vi "young.vi"() -> ()   [LabVIEW 2018]
doc: "Logs and displays weather data in real-time from the Vaisala WXT520 Weather Station and the Optical Scientific ORG-815 Optical Rain Gauge."
uses:
  <vilib>/Analysis/baseanly.llb/Mean (DBL).vi
  <vilib>/Platform/browser.llb/Open URL in Default Browser (path).vi
  <vilib>/Analysis/NI_AALBase.lvlib
panel:
  out "Wind Gusts":dbl format="%.3g"
  out "RF Propagation Logo":picture
  in  "Show Legend":bool
  out "Young Logo":picture
  in  "Young Prefix":string="Young"
  in  "Young":refnum<visa-resource-name>="Port3"
  out "Date":string="2012/06/22\n12:33:20 PM"
  out "Wind Direction":dbl format="%.3g"
  out "Wind Speed":dbl format="%.3g"
  out "Pressure":dbl format="%.3g"
  out "Humidity":dbl format="%.3g"
  out "Temperature":dbl format="%.3g"
  in  "Open Output":bool
  out "Running LED":bool
  out "Uptime":string="00:00:00"
  out "Progress Bar":u32(slide) scale=0.0..60.0
  in  "stop":bool
  out "Timestamp":dbl
  in  "Output Path":path=path "C:/Users/Bruce Wayne/Desktop/DELETE_WeatherTest"
  out "Rain Fall":dbl format="%.3g"
  out "Rain Rate":dbl format="%.3g"
  out "Header":picture
  out "SCaN Logo":picture
  out "NASA Logo":picture
  out "Warning":string
  out "Plot 3":cluster{"array":dbl[], "array":dbl[]}[](graph)
  out "Plot 2":cluster{"array":dbl[], "array":dbl[]}[](graph)
  out "Plot 1":cluster{"array":dbl[], "array":dbl[]}[](graph)
  out "Young Error":bool
  out "Legend":picture
  out "Young":T1
  # "Port"
  # "File Prefix"
  # "seconds"
  # "CONDITIONS"
  # "mm / hr"
  # "mm"
  # "°C"
  # "%"
  # "mBar"
  # "m / s"
  # "°"
  # "m / s"
  # "Recording"
  # "Version 2.0\nNASA Glenn Research Center\nmichael.j.zemba@nasa.gov"
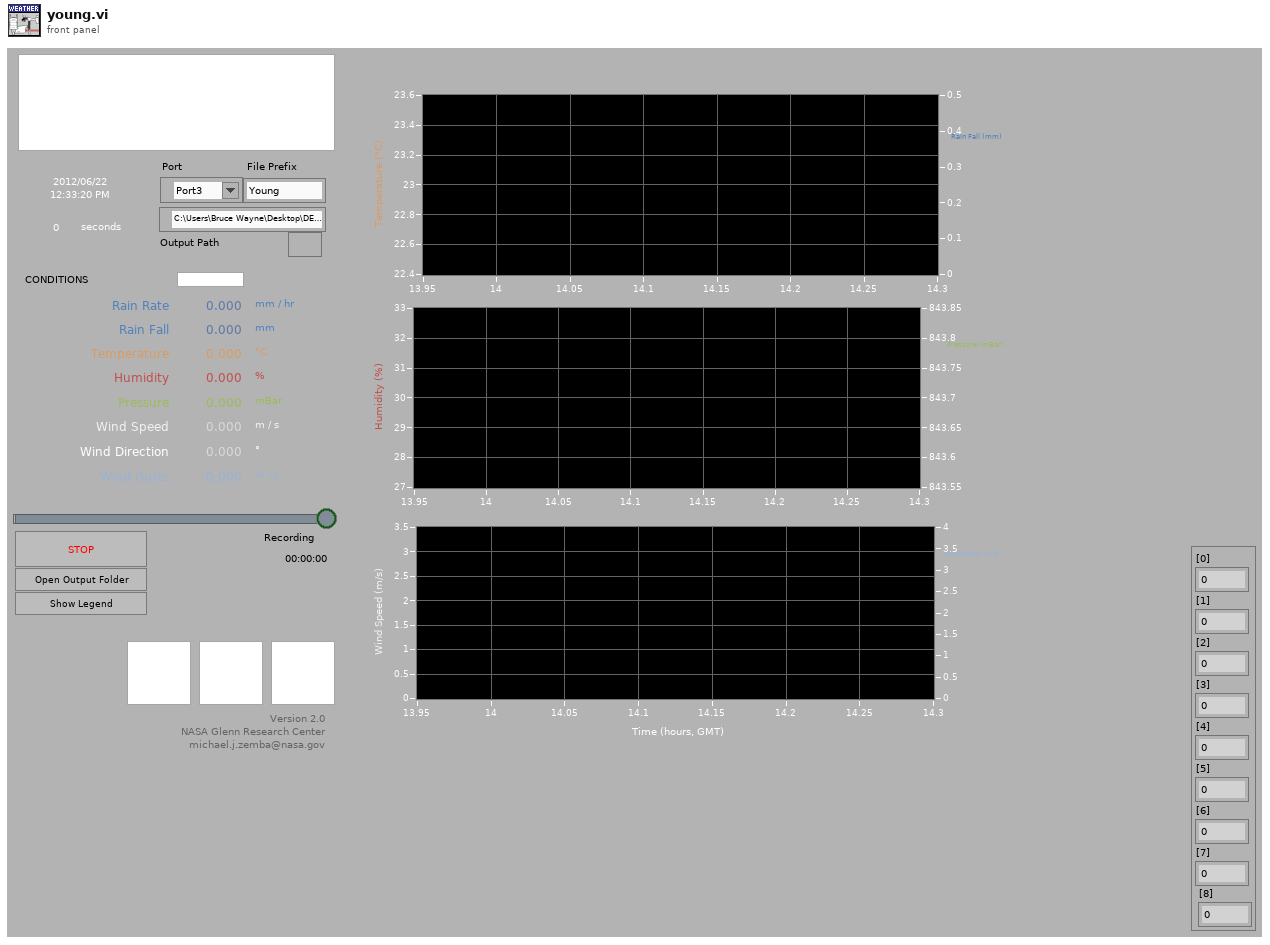
[diagram p1: front panel]
types:
  T1 = cluster{"[0]":dbl, "[1]":dbl, "[2]":dbl, "[3]":dbl, "[4]":dbl, "[5]":dbl, "[6]":dbl, "[7]":dbl, "[8]":dbl}
  T2 = cluster{"Timestamp":dbl[], "ORG Rain Fall":dbl[]}[]
  T3 = cluster{"Timestamp":dbl[], "WXT Pressure":dbl[]}[]
  T4 = cluster{"Timestamp":dbl[], "WXT Wind Direction":dbl[]}[]
  T5 = cluster{"[0]":dbl, "[1]":dbl, "[2]":dbl, "[3]":dbl, "[4]":dbl, "[5]":dbl, "[6]":dbl, "[7]":dbl}
  T6 = cluster{"[0]":dbl, dbl, "[1]":dbl, "[2]":dbl, "[3]":dbl, "[4]":dbl, dbl, "[6]":dbl, dbl}
  T7 = typedef "imagedata.ctl" = cluster{"image type":i32, "image depth":i32, "image":u8[], "mask":u8[], "colors":u32[], "Rectangle":cluster{"left":i16, "top":i16, "right":i16, "bottom":i16}}
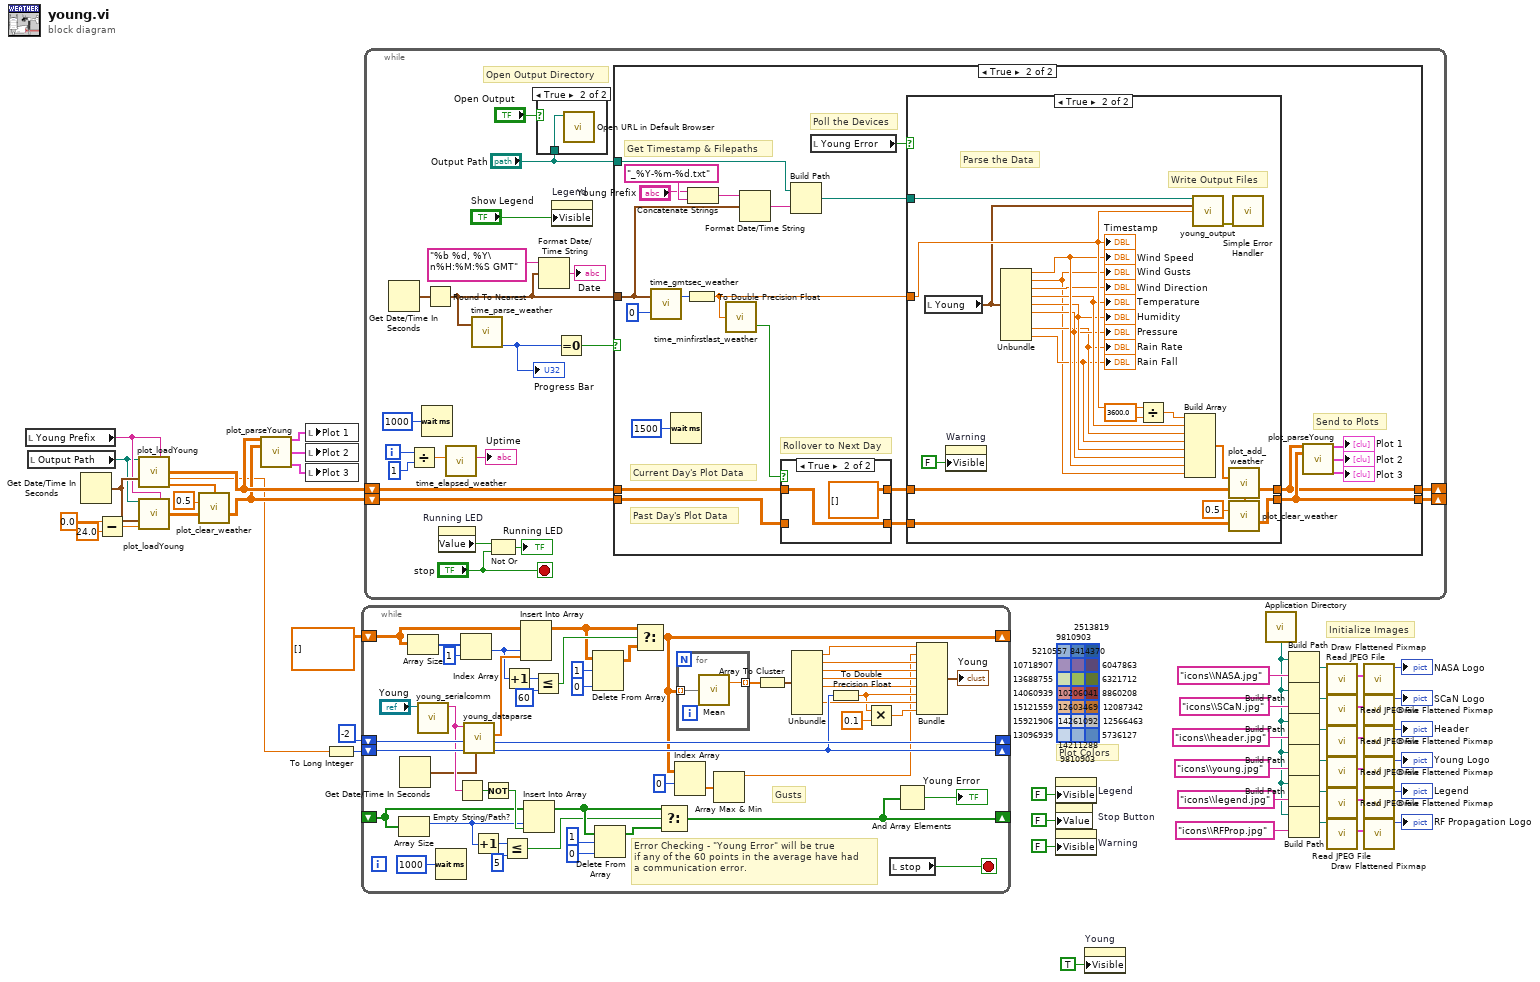
[diagram p0: block diagram]
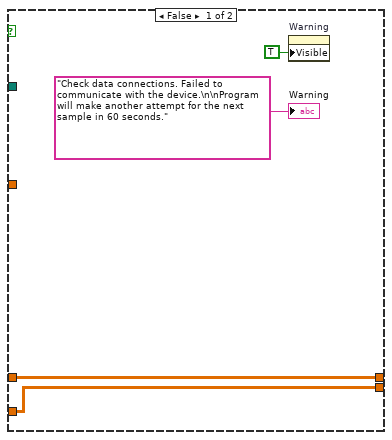
[diagram p4: hidden frame]
diagram:
  (unwired) u32 6321712
  (unwired) u32 8860208
  (unwired) u32 12087342
  (unwired) u32 12566463
  (unwired) u32 5736127
  (unwired) u32 14060939
  (unwired) u32 15121559
  (unwired) u32 15921906
  (unwired) u32 13096939
  (unwired) u32 13688755
  (unwired) u32 6047863
  (unwired) u32 10718907
  (unwired) u32 9810903
  (unwired) u32 10206041
  (unwired) u32 8414370
  (unwired) u32 12603469
  (unwired) u32 14261092
  (unwired) u32 14211288
  (unwired) u32 9810903
  (unwired) u32 2513819
  (unwired) u32 5210557
  # "Plot Colors"
  # "Initialize Images"
  n1 = local read "Young Prefix"() -> (w13:string)
  n2 = local read "Output Path"() -> (w3:path)
  n3 = Get Date/Time In Seconds() -> (seconds since 1Jan1904=w17:timestamp)
  n4 = Subtract(x=0.0, y=24.0) -> (x-y=w14:dbl)
  n5 = call "plot_loadYoung.vi"("Output Path"=w3, "Young Prefix"=w13, "Time"=w17) -> ("Loaded Data Array"=w9:dbl[][], "Last Tips Value"=w2:dbl, "Timestamp"=w12:dbl[])  [unwired: 10 in]
  n6 = call "plot_loadYoung.vi"("Output Path"=w3, "Young Prefix"=w13, "Time"=w17, "Offset (hrs)"=w14) -> ("Loaded Data Array"=w11:dbl[][])  [unwired: 9 in, 2 out]
  n7 = call "plot_clear_weather.vi"("Clearing Array"=w12, "Buffer Size"=0.5, "Input Arrays"=w11) -> ("Output Arrays"=w8:dbl[][])  [unwired: 12 in]
  n8 = call "plot_parseYoung.vi"("Current Data"=w9, "Yesterday's Data"=w8) -> ("Plot 1"=w6:T2, "Plot 2"=w7:T3, "Plot 3"=w5:T4)  [unwired: 11 in]
  n9 = local write "Plot 1"(w6) -> ()
  n10 = local write "Plot 2"(w7) -> ()
  n11 = local write "Plot 3"(w5) -> ()
  n12 = To Long Integer(number=w2) -> (32bit integer=w4:i32)
  n13 = while {
    shift-right: [w95] -> _
    shift-left: -2 ("TB Out") -> [w97]
    shift-right: [w75] -> _
    shift-left: w4 -> [w96]
    shift-right: [w59] -> _
    shift-left: dbl[][] [] ("Plot Arrays") -> [w93]
    shift-right: [w64] -> _
    shift-left: _ -> [w71]
    stop <- w80 stop-if-true
    # "Gusts"
    # "Error Checking - \"Young Error\" will be true\nif any of the 60 points in the average have had\na communication error."
    n14 = Array Size(array=w71) -> (size(s)=w69:i32)
    n15 = Get Date/Time In Seconds() -> (seconds since 1Jan1904=w60:timestamp)
    n16 = Array Size(array=w93) -> (size(s)=w92:i32[])
    n17 = call "young_serialcomm.vi"("Resource Name"="Young") -> ("Poll Response"=w73:string)  [unwired: 8 in, 2 out]
    n18 = Wait (ms)(milliseconds to wait=u32 1000) -> ()  [unwired: 1 out]
    n19 = Empty String/Path?(string/path=w73) -> (empty?=w74:bool)
    n20 = Index Array(array=w92, index=1) -> (element=w90:i32)
    n21 = call "young_dataparse.vi"("Current Time"=w60, "Tips In"=w96, "TB In"=w97, "Poll Response"=w73) -> ("Tips Out"=w75:i32, "TB Out"=w95:i32, "Output Array"=w94:dbl[])  [unwired: 5 in]
    n22 = Increment(x=w69) -> (x+1=w70:i32)
    n23 = Not(x=w74) -> (.not. x?=w72:bool)
    n24 = Less Or Equal?(x=w70, y=5) -> (x <= y?=w65:bool)
    n25 = Increment(x=w90) -> (x+1=w89:i32)
    n26 = Insert Into Array(array=w93, index (col)=w90, new element=w94) -> (w86:dbl[][])  [unwired: 1 in]
    n27 = Insert Into Array(array=w71, index=w69, new element=w72) -> (w67:bool[])
    n28 = Less Or Equal?(x=w89, y=60) -> (x <= y?=w87:bool)
    n29 = Delete From Array(array=w86, length=1, index (col)=0 ("disabled index (col)")) -> (array with subset deleted=w85:dbl[][])  [unwired: 1 in, 1 out]
    n30 = Delete From Array(array=w67, length=1, index=0) -> (array with subset deleted=w66:bool[])  [unwired: 1 out]
    n31 = Select(t=w86, s=w87, f=w85) -> (s? t:f=w59:dbl[][])
    n32 = Select(t=w67, s=w65, f=w66) -> (s? t:f=w64:bool[])
    n33 = Index Array(array=w59, index (row)=0) -> (element=w57:dbl[])  [unwired: 1 in]
    n34 = for {
      tunnel: w59 -> [w99] mode=indexing
      tunnel: [w98] -> w81 mode=indexing
      n35 = call-poly <vilib>:"Mean.vi"("X"=w99) -> ("mean"=w98:dbl)  [unwired: 1 out]
    }
    n36 = Array Max & Min(array=w57) -> (max value=w49:dbl)  [unwired: 3 out]
    n37 = Array To Cluster(array=w81) -> (cluster=w78:T5)
    n38 = Unbundle(w78) -> ("[0]"=w77:dbl, "[1]"=w50:dbl, "[2]"=w51:dbl, "[3]"=w52:dbl, "[4]"=w53:dbl, "[6]"=w55:dbl)  [unwired: 2 out]
    n39 = To Double Precision Float(number=w75) -> (double precision float=w54:dbl)
    n40 = Multiply(x=w54, y=0.1) -> (x*y=w56:dbl)
    n41 = local read "stop"() -> (w80:bool)
    n42 = And Array Elements(Boolean array=w64) -> (logical AND=→"Young Error":bool)
    n43 = Bundle("[0]"=w77, w49, "[1]"=w50, "[2]"=w51, "[3]"=w52, "[4]"=w53, w54, "[6]"=w55, w56) -> (→"Young":T6)  [unwired: 1 in]
  }
  n44 = while {
    shift-right: [w112] -> _
    shift-left: w9 -> [w111]
    shift-right: [w109] -> _
    shift-left: w8 -> [w110]
    i -> [w103]
    stop <- "stop" stop-if-true
    # "Open Output Directory"
    n45 = Get Date/Time In Seconds() -> (seconds since 1Jan1904=w101:timestamp)
    n46 = Divide(x=w103, y=1) -> (x/y=w104:dbl)
    n47 = Wait (ms)(milliseconds to wait=u32 1000) -> ()  [unwired: 1 out]
    n48 = Round To Nearest(number=w101) -> (nearest integer value=w100:timestamp)
    n49 = property on="Running LED" class="Bool (strict)"() -> ("Value"=w120:bool)  [unwired: 2 in, 2 out]
    n50 = call "time_elapsed_weather.vi"("Elapsed Time (sec)"=w104) -> ("Elapsed Time (string)"=→"Uptime":string)  [unwired: 10 in]
    n51 = call "time_parse_weather.vi"("Current Time"=w100) -> ("Seconds"=w105:u32)  [unwired: 12 in, 6 out]
    "Progress Bar" <- w105
    n52 = Not Or(1:"stop", 2:w120) -> (0:→"Running LED":bool)
    n53 = case shown="True" "Open Output" {
      tunnel: "Output Path" -> [_ w121]
      frame False {
      }
      frame True {
        n54 = call-poly <vilib>:"Open URL in Default Browser.vi"("path"=w121) -> ()  [unwired: 5 in, 2 out]
      }
    }
    n55 = Format Date/Time String(time format string (%c)="%b %d, %Y\n%H:%M:%S GMT", seconds (now)=w100) -> (date/time string=→"Date":string)  [unwired: 1 in]
    n56 = property on="Legend" class="Pict"("Visible"="Show Legend") -> ()  [unwired: 2 in, 2 out]
    n57 = Equal To 0?(x=w105) -> (x = 0?=w118:bool)
    n58 = case shown="True" w118 {
      tunnel: "Output Path" -> [_ w142]
      tunnel: w100 -> [_ w128]
      tunnel: [w123 w130] -> w112
      tunnel: w111 -> [w123 w145]
      tunnel: w110 -> [w122 w144]
      tunnel: [w122 w131] -> w109
      frame False {
      }
      frame True {
        # "Send to Plots"
        # "Current Day's Plot Data"
        # "Past Day's Plot Data"
        # "Poll the Devices"
        # "Rollover to Next Day"
        # "Get Timestamp & Filepaths"
        n59 = call "time_gmtsec_weather.vi"("Timezone Offset (Hrs)"=0, "Timestamp"=w128) -> ("Sec Since 12AM GMT"=w126:u32)  [unwired: 1 out]
        n60 = Wait (ms)(milliseconds to wait=u32 1500) -> ()  [unwired: 1 out]
        n61 = To Double Precision Float(number=w126) -> (double precision float=w125:dbl)
        n62 = Concatenate Strings("Young Prefix", "_%Y-%m-%d.txt" ("string")) -> (w139:string)
        n63 = call "time_minfirstlast_weather.vi"("Sec. from Midnight"=w125) -> ("First Minute of Day"=w135:bool)  [unwired: 2 in, 1 out]
        n64 = Format Date/Time String(time format string (%c)=w139, seconds (now)=w128) -> (date/time string=w143:string)  [unwired: 1 in]
        n65 = case shown="True" w135 {
          tunnel: w145 -> [w173 w175]
          tunnel: [w173 dbl[][] [] ("Input Arrays")] -> w137
          tunnel: [w172 w175] -> w136
          tunnel: w144 -> [w172 _]
          frame False {
          }
          frame True {
          }
        }
        n66 = Build Path(base path=w142, name or relative path=w143) -> (appended path=w138:path)
        n67 = local read "Young Error"() -> (w129:bool)
        n68 = case shown="True" w129 {
          tunnel: w125 -> [_ w164]
          tunnel: w138 -> [_ w161]
          tunnel: w137 -> [w149 w167]
          tunnel: [w149 w166] -> w130
          tunnel: w136 -> [w148 w168]
          tunnel: [w148 w165] -> w131
          frame False {
            n69 = property on="Warning" class="Str"("Visible"=TRUE) -> ()  [unwired: 2 in, 2 out]
            "Warning" <- "Check data connections. Failed to communicate with the device.\n\nProgram will make another attempt for the next sample in 60 seconds."
          }
          frame True {
            # "Parse the Data"
            # "Write Output Files"
            n70 = local read "Young"() -> (w151:T1)
            n71 = property on="Warning" class="Str"("Visible"=FALSE) -> ()  [unwired: 2 in, 2 out]
            n72 = Unbundle(w151) -> ("[0]"=w158:dbl, "[1]"=w150:dbl, "[2]"=→"Wind Direction":dbl, "[3]"=w156:dbl, "[4]"=w155:dbl, "[5]"=w154:dbl, "[7]"=w153:dbl, "[8]"=w152:dbl)  [unwired: 1 out]
            "Rain Rate" <- w153
            "Rain Fall" <- w152
            "Temperature" <- w156
            "Humidity" <- w155
            "Pressure" <- w154
            "Wind Speed" <- w158
            "Wind Gusts" <- w150
            n73 = Divide(x=w164, y=3600.0) -> (x/y=w163:dbl)
            n74 = Build Array(w163, w156, w153, w152, w155, w154, w158, w150) -> (w169:dbl[])
            n75 = call "young_output.vi"("Output Path"=w161, "YOUNG  Data Cluster"=w151, "Timestamp"=w164) -> ("Error Out"=w159:errorcluster)  [unwired: 12 in]
            n76 = call "plot_add_weather.vi"("Input Points"=w169, "Input Arrays"=w167) -> ("Output Arrays"=w166:dbl[][], "Timestamps"=w171:dbl[])  [unwired: 12 in]
            n77 = call "plot_clear_weather.vi"("Clearing Array"=w171, "Buffer Size"=0.5, "Input Arrays"=w168) -> ("Output Arrays"=w165:dbl[][])  [unwired: 12 in]
            n78 = call <vilib>:"Simple Error Handler.vi"("error in (no error)"=w159) -> ()  [unwired: 1 in, 8 out]
            "Timestamp" <- w164
          }
        }
        n79 = call "plot_parseYoung.vi"("Current Data"=w130, "Yesterday's Data"=w131) -> ("Plot 1"=→"Plot 1":T2, "Plot 2"=→"Plot 2":T3, "Plot 3"=→"Plot 3":T4)  [unwired: 11 in]
      }
    }
  }
  n80 = property on="Legend" class="Pict"("Visible"=FALSE) -> ()  [unwired: 2 in, 2 out]
  n81 = property on="Stop Button" class="Bool (strict)"("Value"=FALSE ("Visible")) -> ()  [unwired: 2 in, 2 out]
  n82 = property on="Warning" class="Str"("Visible"=FALSE) -> ()  [unwired: 2 in, 2 out]
  n83 = property on="Young" class="Clust (strict)"("Visible"=TRUE) -> ()  [unwired: 2 in, 2 out]
  n84 = call <vilib>:"Application Directory.vi"() -> ("Application Directory"=w19:path)
  n85 = Build Path(base path=w19, name or relative path="icons\\NASA.jpg") -> (appended path=w39:path)
  n86 = Build Path(base path=w19, name or relative path="icons\\SCaN.jpg") -> (appended path=w38:path)
  n87 = Build Path(base path=w19, name or relative path="icons\\header.jpg") -> (appended path=w37:path)
  n88 = Build Path(base path=w19, name or relative path="icons\\young.jpg") -> (appended path=w35:path)
  n89 = Build Path(base path=w19, name or relative path="icons\\legend.jpg") -> (appended path=w24:path)
  n90 = Build Path(base path=w19, name or relative path="icons\\RFProp.jpg") -> (appended path=w22:path)
  n91 = call <vilib>:"Read JPEG File.vi"("path to JPEG file"=w39) -> ("image data"=w46:T7)  [unwired: 8 in, 2 out]
  n92 = call <vilib>:"Read JPEG File.vi"("path to JPEG file"=w38) -> ("image data"=w45:T7)  [unwired: 8 in, 2 out]
  n93 = call <vilib>:"Read JPEG File.vi"("path to JPEG file"=w37) -> ("image data"=w44:T7)  [unwired: 8 in, 2 out]
  n94 = call <vilib>:"Read JPEG File.vi"("path to JPEG file"=w35) -> ("image data"=w33:T7)  [unwired: 8 in, 2 out]
  n95 = call <vilib>:"Read JPEG File.vi"("path to JPEG file"=w24) -> ("image data"=w28:T7)  [unwired: 8 in, 2 out]
  n96 = call <vilib>:"Read JPEG File.vi"("path to JPEG file"=w22) -> ("image data"=w21:T7)  [unwired: 8 in, 2 out]
  n97 = call <vilib>:"Draw Flattened Pixmap.vi"("image data"=w46) -> ("new picture"=→"NASA Logo":picture)  [unwired: 8 in]
  n98 = call <vilib>:"Draw Flattened Pixmap.vi"("image data"=w45) -> ("new picture"=→"SCaN Logo":picture)  [unwired: 8 in]
  n99 = call <vilib>:"Draw Flattened Pixmap.vi"("image data"=w44) -> ("new picture"=→"Header":picture)  [unwired: 8 in]
  n100 = call <vilib>:"Draw Flattened Pixmap.vi"("image data"=w33) -> ("new picture"=→"Young Logo":picture)  [unwired: 8 in]
  n101 = call <vilib>:"Draw Flattened Pixmap.vi"("image data"=w28) -> ("new picture"=→"Legend":picture)  [unwired: 8 in]
  n102 = call <vilib>:"Draw Flattened Pixmap.vi"("image data"=w21) -> ("new picture"=→"RF Propagation Logo":picture)  [unwired: 8 in]
